vi "receta.vi"() -> ()   [LabVIEW 2025]
uses:
  <vilib>/Instr/_visa.llb/VISA Configure Serial Port (Instr).vi
panel:
  in  "VISA resource name":refnum<visa-resource-name>
  out "String":string
  in  "stop":bool
  in  "PANCAKES":bool
  in  "BANANO":bool
  in  "CHOCOLO":bool
  # "Selecciona tu receta"
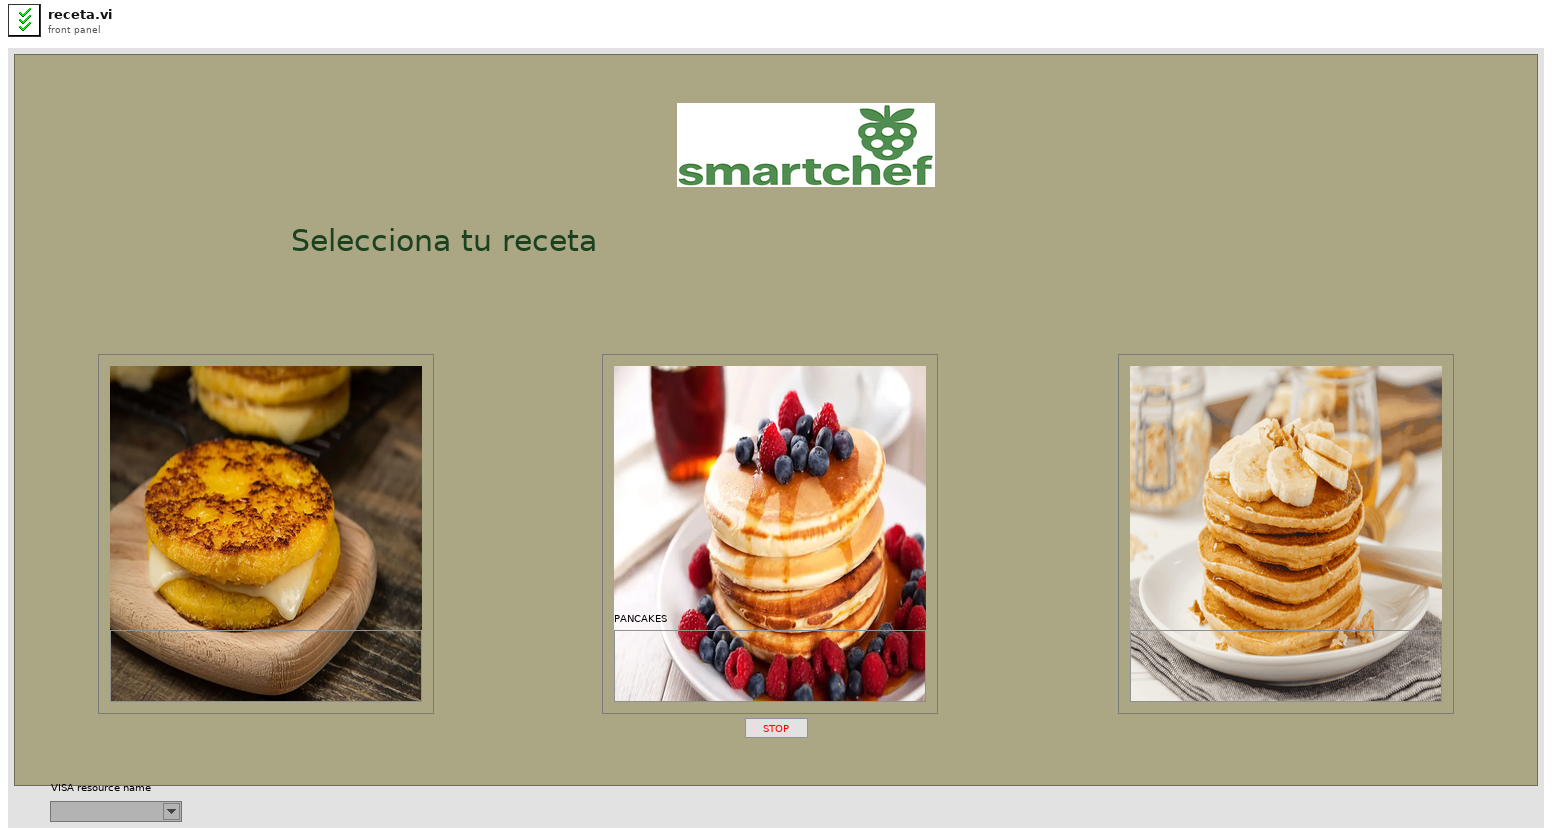
[diagram p1: front panel]
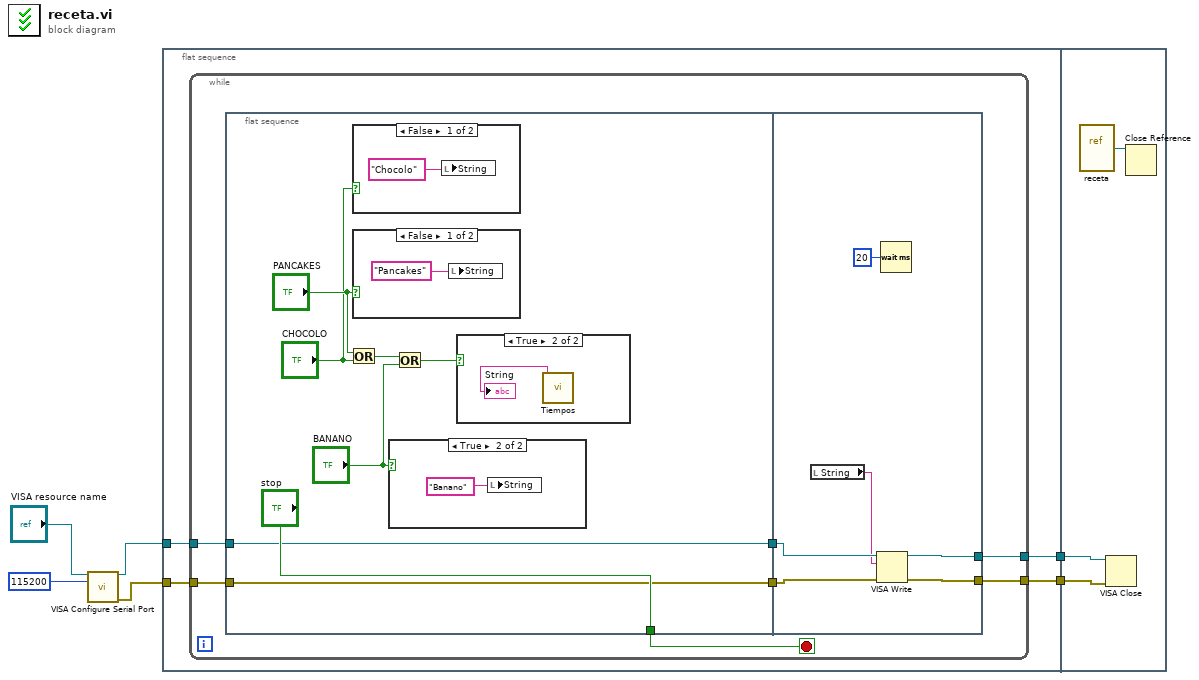
[diagram p0: block diagram]
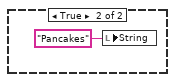
[diagram p4: hidden frame]
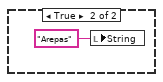
[diagram p5: hidden frame]
diagram:
  n1 = call-poly "VISA Configure Serial Port"("VISA resource name"="VISA resource name", "baud rate (9600)"=u32 115200) -> ("VISA resource name out"=w4:refnum<visa-resource-name>, "error out"=w3:errorcluster)  [unwired: 12 in]
  n2 = flat-sequence {
    tunnel: w4 -> [w10]
    tunnel: w3 -> [w9]
    tunnel: [w8] -> w2
    tunnel: [w7] -> w1
    tunnel: w2 -> [w39]
    tunnel: w1 -> [w38]
    frame #0 {
      n3 = while {
        tunnel: w10 -> [w15]
        tunnel: w9 -> [w13]
        tunnel: [w12] -> w8
        tunnel: [w11] -> w7
        stop <- w17 stop-if-true
        n4 = flat-sequence {
          tunnel: ["stop"] -> w17
          tunnel: [w19] -> w16
          tunnel: w15 -> [w19]
          tunnel: [w18] -> w14
          tunnel: w13 -> [w18]
          tunnel: w16 -> [w37]
          tunnel: w14 -> [w36]
          tunnel: [w35] -> w12
          tunnel: [w34] -> w11
          frame #0 {
            n5 = Or(x="PANCAKES", y="CHOCOLO") -> (x .or. y?=w22:bool)
            n6 = case shown="False" "CHOCOLO" {
              frame False {
                n7 = local write "String"("Chocolo") -> ()
              }
              frame True {
                n8 = local write "String"("Arepas") -> ()
              }
            }
            n9 = case shown="False" "PANCAKES" {
              frame False {
                n10 = local write "String"("Pancakes") -> ()
              }
              frame True {
                n11 = local write "String"("Pancakes") -> ()
              }
            }
            n12 = case shown="True" "BANANO" {
              frame False {
              }
              frame True {
                n13 = local write "String"("Banano") -> ()
              }
            }
            n14 = Or(x=w22, y="BANANO") -> (x .or. y?=w20:bool)
            n15 = case shown="True" w20 {
              frame False {
              }
              frame True {
                n16 = call "Tiempos.vi"() -> ("RECETA"=→"String":string)  [unwired: 3 in]
              }
            }
          }
          frame #1 {
            n17 = local read "String"() -> (w33:string)
            n18 = VISA Write(VISA resource name=w37, write buffer=w33, error in (no error)=w36) -> (VISA resource name out=w35:refnum<visa-resource-name>, error out=w34:errorcluster)  [unwired: 1 out]
            n19 = Wait (ms)(milliseconds to wait=u32 20) -> ()  [unwired: 1 out]
          }
        }
      }
    }
    frame #1 {
      n20 = vi-ref "receta.vi"() -> (w40:refnum<vi>)
      n21 = VISA Close(VISA resource name=w39, error in (no error)=w38) -> ()  [unwired: 1 out]
      n22 = Close Reference(reference=w40) -> ()  [unwired: 1 in, 1 out]
    }
  }
